vi "Show_Image.vi"(8 "error in (no error)":errorcluster, 11 ".NET Refnum In":refnum<k24>) -> (0 "error out":errorcluster, 1 "u8Image":u8[](array[numeric]), 2 "Image":picture, 3 ".NET Refnum Out":refnum<k24>)   [LabVIEW 2021]
uses:
  C:/Program Files/Thorlabs/Scientific Imaging/ThorCam/uc480DotNet.dll
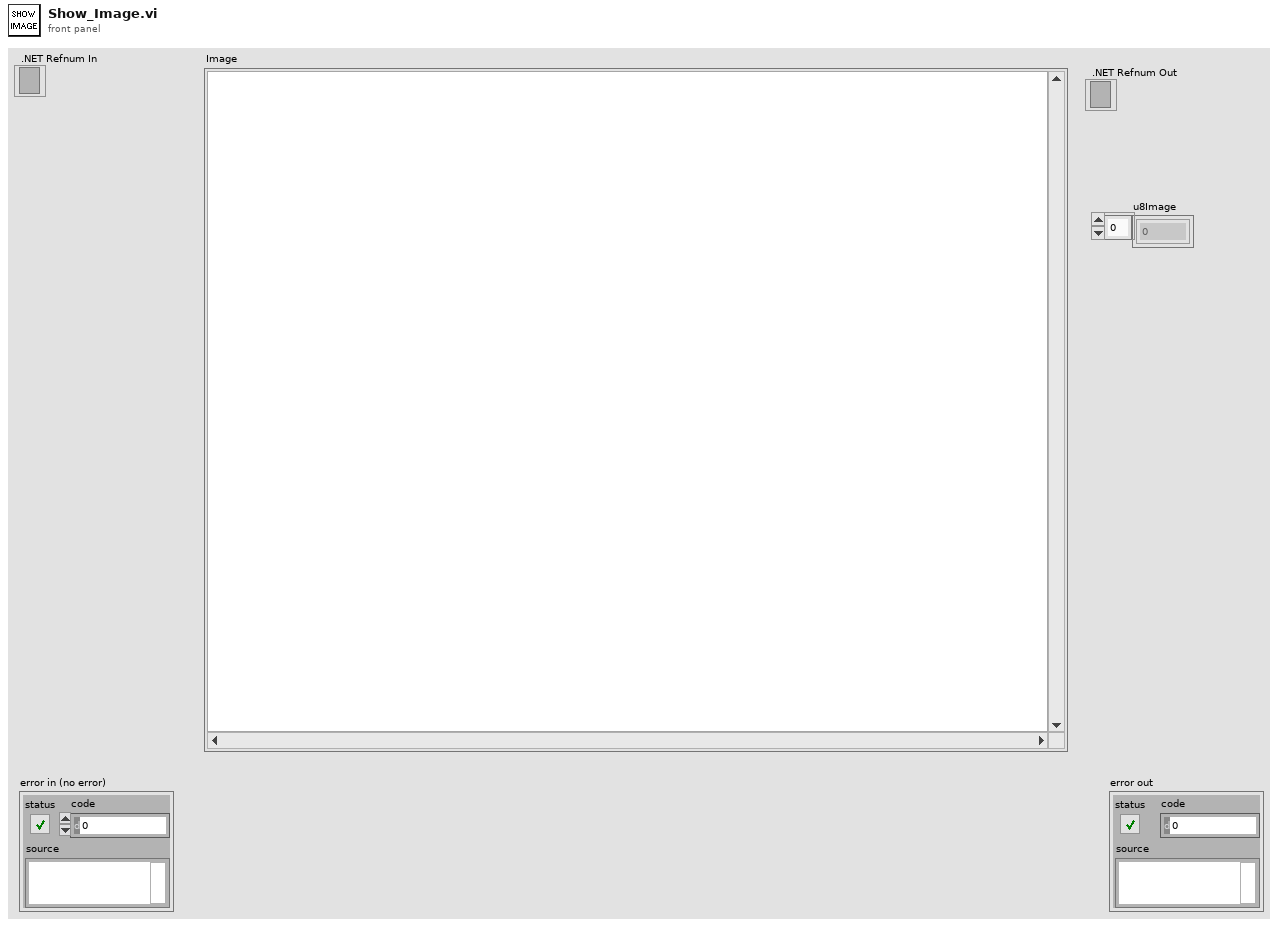
[diagram p1: front panel]
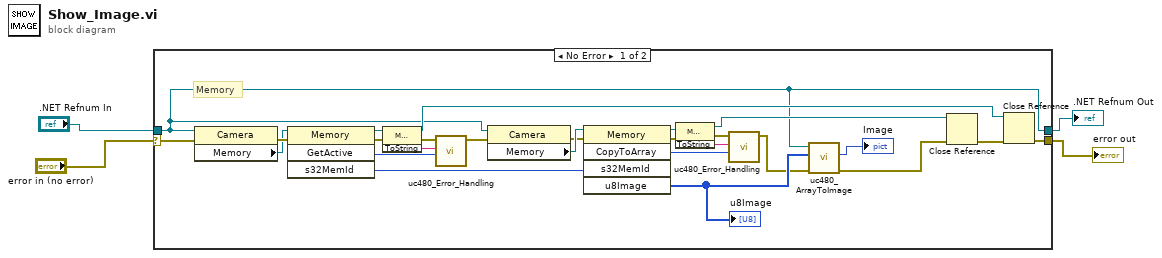
[diagram p0: block diagram]
diagram:
  n1 = case shown="No Error" "error in (no error)" {
    selector: "error in (no error)" -> [w6 w32]
    tunnel: [w26 w32] -> w4
    tunnel: ".NET Refnum In" -> [w5 w31]
    tunnel: [w5 w31] -> w1
    frame No Error {
      # "Memory"
      n2 = property class="Camera"(reference=w5, error in=w6) -> (error out=w21:errorcluster, "Memory"=w20:refnum<k24>)  [unwired: 1 out]
      n3 = invoke class="Memory" method="GetActive"(reference=w20, error in=w21) -> (reference out=w14:refnum<k24>, error out=w15:errorcluster, "GetActive"=w13:i32, "s32MemId"=w22:i32)  [unwired: 2 in]
      n4 = invoke class="Memory" method="ToString"(reference=w14, error in=w15) -> (reference out=w27:refnum<k24>, error out=w17:errorcluster, "ToString"=w16:string)  [unwired: 1 in]
      n5 = call "uc480_Error_Handling.vi"("Error Code"=w13, "Error String"=w16, "Error In"=w17) -> ("Error Out"=w12:errorcluster)  [unwired: 8 in]
      n6 = property class="Camera"(reference=w5, error in=w12) -> (error out=w18:errorcluster, "Memory"=w19:refnum<k24>)  [unwired: 1 out]
      n7 = invoke class="Memory" method="CopyToArray"(reference=w19, error in=w18, "s32MemId"=w22) -> (reference out=w9:refnum<k24>, error out=w8:errorcluster, "CopyToArray"=w7:i32, "u8Image"=w25:u8[])  [unwired: 2 in, 1 out]
      "u8Image" <- w25
      n8 = invoke class="Memory" method="ToString"(reference=w9, error in=w8) -> (reference out=w30:refnum<k24>, error out=w11:errorcluster, "ToString"=w10:string)  [unwired: 1 in]
      n9 = call "uc480_Error_Handling.vi"("Error Code"=w7, "Error String"=w10, "Error In"=w11) -> ("Error Out"=w24:errorcluster)  [unwired: 8 in]
      n10 = call "uc480_ArrayToImage.vi"("Error In"=w24, "InArray"=w25, "uc480.Camera"=w5) -> ("Error Out"=w29:errorcluster, "Image"=→"Image":picture)  [unwired: 7 in]
      n11 = Close Reference(reference=w30, error in (no error)=w29) -> (error out=w28:errorcluster)
      n12 = Close Reference(reference=w27, error in (no error)=w28) -> (error out=w26:errorcluster)
    }
    frame Error {
    }
  }
  "error out" <- w4
  ".NET Refnum Out" <- w1
